vi "Create GB by Co-incident O-lattice.vi"(5 "Skip cleanup?":bool, 6 "Max # of atoms":i32=9999999, 7 "Collision Removal":T1={"Min Seperation Distance (A)"=2.0, "Edge Duplication Range (A)"=3.0}, 8 "Co-incident Tolerance":dbl=0.01, 9 "Number of integers to search":i32=50, 10 "Grain Growth and Geometry":T5={"Min Grain Length (A)"=5.0, "Min Angle from GB plane"=0.0, "GB Overlap Length (A)"=0.0}, 11 "Grain Boundary Definition":T6={"Grain 1 Orientation"=[1.0, 0.6019417241891012, 0.029651947654046266], "Grain 2 Orientation"=[1.0, 0.730727623275494, 0.2205637301176], "Twist Angle (Deg)"=0.0, "Translation Vector"=[0.0, 0.0, 0.0]}) -> (1 "Creation Time":T4={"Time to create primitives"=0, "Time to Grow to Box"=4152, "Time to find subset"=1109, "Time to Cleanup"=1}, 2 "GB Data":string[][](array[string])=[["Grain 1, h", "Grain 1, k", "Grain 1, L", "Grain 2, h", "Grain 2, k", "Grain 2, L", "Twist Angle (Deg)", "Translation Tx", "Translation Ty", "Translation Tz", "Tilt Angle (Deg)", "Viewing Angle, h", "Viewing Angle, k", "Viewing Angle, L", "Grain 1 Length (factor)", "Grain 2 Length (factor", "Max Grain Height (A)", "Max Grain Width (A)", "Grain 1 Start", "Overlap Region (A)", "Reduction Slab X", "Reduction Slab Y", "Reduction Tolerance (A)", "Min Atomic Separation Distance", "Edge Duplication Range", "# Atoms"], ["1.000000", "0.601942", "0.029652", "1.000000", "0.730728", "0.220564", "0.000000", "0.000000", "0.000000", "0.000000", "10.024930", "1.000000", "-1.661290", "0.000000", "1.000000", "1.000000", "90.000000", "90.000000", "-0.001000", "0.001000", "4.600000", "4.000000", "0.500000", "2.000000", "3.000000", "12135.000000"]], 3 "Grain Boundary":T2={"Structure Name"="(0.00) twist [1.000,0.602,0.030] [1.000,0.731,0.221] (0.00,0.00,0.00)T GB", "Lattice vector a"=[270.03, 0.0, 0.0], "Lattice vector b"=[0.0, 270.03, 0.0], "Lattice vector c"=[0.0, 0.0, 6.006], "Atoms Array"=[{"Atom Name"="Cd", "Positions (Direct)"=array6055x3[18165 elements], "Positions (Cartesian)"=array6055x3[18165 elements]}, {"Atom Name"="Te", "Positions (Direct)"=array6080x3[18240 elements], "Positions (Cartesian)"=array6080x3[18240 elements]}], "# of atoms"=12135} {"Atoms Array"."Positions (Cartesian)" format="%#_4f"; "Atoms Array"."Positions (Direct)" format="%#_4f"})   [LabVIEW 2010]
uses:
  <vilib>/Analysis/baseanly.llb/Real A x B.vi
  <vilib>/Analysis/NI_AALPro.lvlib
  <vilib>/Analysis/NI_AALBase.lvlib
panel:
  in  "GB Plane 1, Lattice a":dbl[](array[numeric])
  in  "GB Plane 2, Lattice b":dbl[](array[numeric])
  in  "Perpendicular to GB Plane, Lattice c":dbl[](array[numeric])
  in  "Conventional Unit Cell":T2={"Structure Name"="CdTe", "Lattice vector a"=[6.615785553057252, 0.0, 0.0], "Lattice vector b"=[0.0, 6.615785553057252, 0.0], "Lattice vector c"=[0.0, 0.0, 6.615785553057252], "Atoms Array"=[{"Atom Name"="Cd", "Positions (Direct)"=[[0.0, 0.0, 0.0], [0.0, 0.5, 0.5], [0.5, 0.0, 0.5], [0.5, 0.5, 0.0]], "Positions (Cartesian)"=[[0.0, 0.0, 0.0], [0.0, 3.307892776528626, 3.307892776528626], [3.307892776528626, 0.0, 3.307892776528626], [3.307892776528626, 3.307892776528626, 0.0]]}, {"Atom Name"="Te", "Positions (Direct)"=[[0.25, 0.25, 0.25], [0.75, 0.75, 0.25], [0.75, 0.25, 0.75], [0.25, 0.75, 0.75]], "Positions (Cartesian)"=[[1.653946388264313, 1.653946388264313, 1.653946388264313], [4.96183916479294, 4.96183916479294, 1.653946388264313], [4.96183916479294, 1.653946388264313, 4.96183916479294], [1.653946388264313, 4.96183916479294, 4.96183916479294]]}], "# of atoms"=8}
  in  "GB Geometry":T3(radio)=enum."Best Triclinic"
  out "error out":errorcluster
  out "Expected # of Atoms":i32=166
  in  "Headers":string[](array[string])=["Grain 1, h", "Grain 1, k", "Grain 1, L", "Grain 2, h", "Grain 2, k", "Grain 2, L", "Twist Angle (Deg)", "Translation Tx", "Translation Ty", "Translation Tz", "Tilt Angle (Deg)", "Viewing Angle, h", "Viewing Angle, k", "Viewing Angle, L", "Grain 1 Length (factor)", "Grain 2 Length (factor", "Max Grain Height (A)", "Max Grain Width (A)", "Grain 1 Start", "Overlap Region (A)", "Reduction Slab X", "Reduction Slab Y", "Reduction Tolerance (A)", "Min Atomic Separation Distance", "Edge Duplication Range", "# Atoms"]
  out "Time to Cleanup":u32=1
  out "Time to find subset":u32=1109
  out "Time to Grow to Box":u32=4152
  out "Time to create primitives":u32
  out "Tilt Angle":dbl=10.024929742348679
  out "# of Atoms Removed":i32=28
  out "Mutual Viewing Angle":dbl[](array[numeric])=[1.0, -1.6612903871170226, 0.0]
  in  "Primitive Unit Cell":T2={"Structure Name"="CdTe", "Lattice vector a"=[6.615785553057252, 0.0, 0.0], "Lattice vector b"=[0.0, 6.615785553057252, 0.0], "Lattice vector c"=[0.0, 0.0, 6.615785553057252], "Atoms Array"=[{"Atom Name"="Cd", "Positions (Direct)"=[[0.0, 0.0, 0.0], [0.0, 0.5, 0.5], [0.5, 0.0, 0.5], [0.5, 0.5, 0.0]], "Positions (Cartesian)"=[[0.0, 0.0, 0.0], [0.0, 3.307892776528626, 3.307892776528626], [3.307892776528626, 0.0, 3.307892776528626], [3.307892776528626, 3.307892776528626, 0.0]]}, {"Atom Name"="Te", "Positions (Direct)"=[[0.25, 0.25, 0.25], [0.75, 0.75, 0.25], [0.75, 0.25, 0.75], [0.25, 0.75, 0.75]], "Positions (Cartesian)"=[[1.653946388264313, 1.653946388264313, 1.653946388264313], [4.96183916479294, 4.96183916479294, 1.653946388264313], [4.96183916479294, 1.653946388264313, 4.96183916479294], [1.653946388264313, 4.96183916479294, 4.96183916479294]]}], "# of atoms"=8}
  # "Remove Collisions"
  # "Primitives"
  # "Grain Growth"
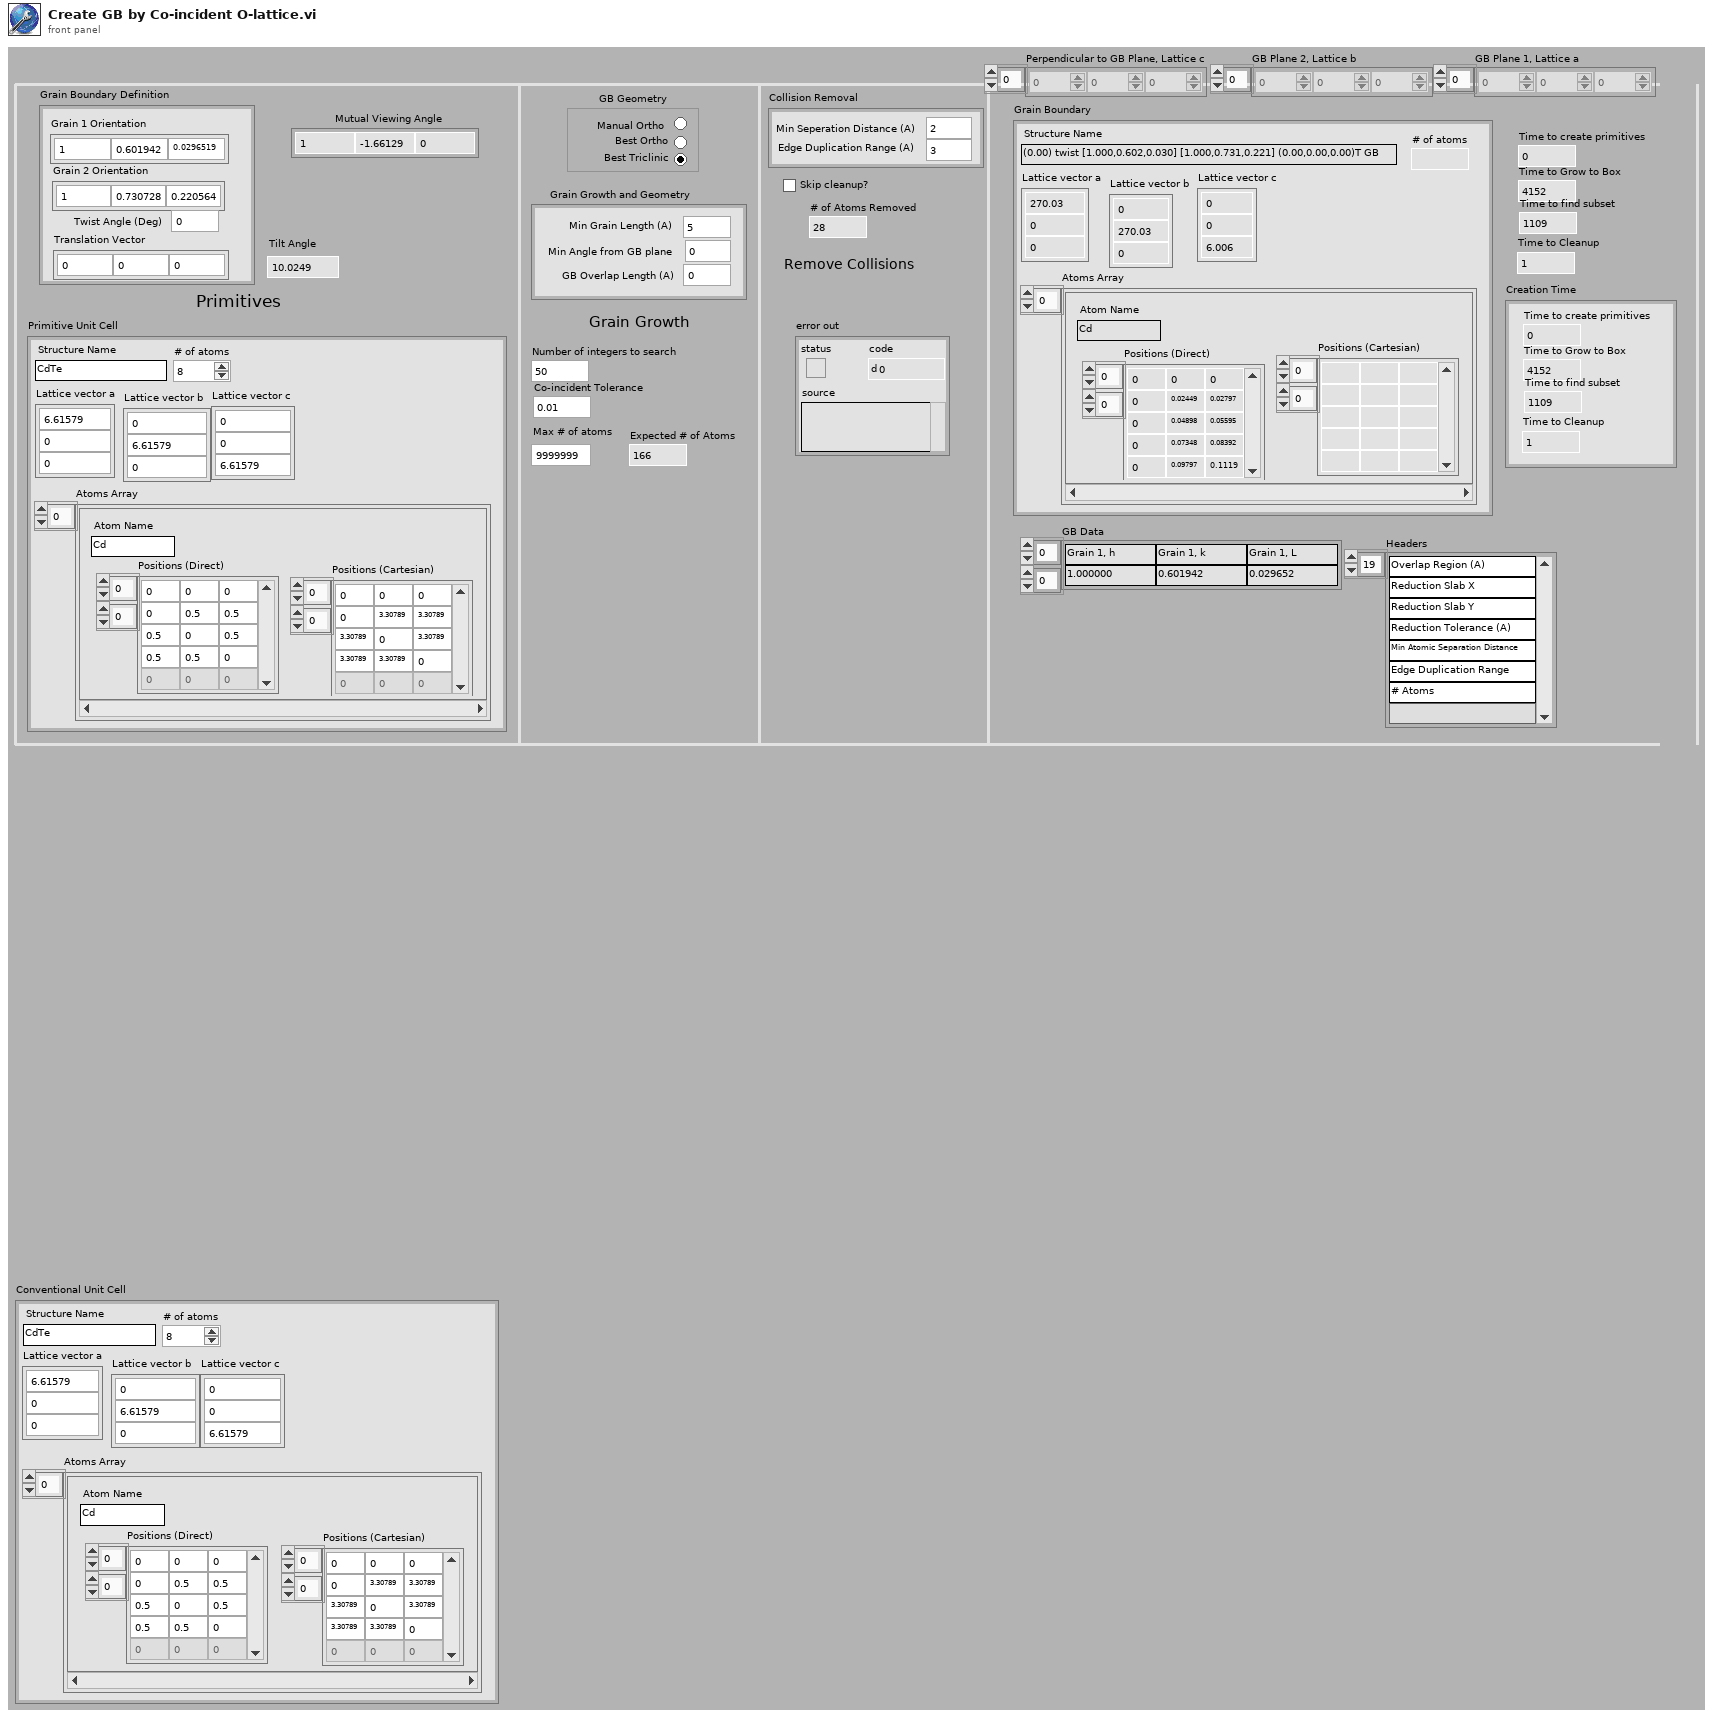
[diagram p1: front panel]
types:
  T1 = cluster{"Min Seperation Distance (A)":dbl, "Edge Duplication Range (A)":dbl}
  T2 = cluster{"Structure Name":string, "Lattice vector a":dbl[], "Lattice vector b":dbl[], "Lattice vector c":dbl[], "Atoms Array":cluster{"Atom Name":string, "Positions (Direct)":dbl[][], "Positions (Cartesian)":dbl[][]}[], "# of atoms":i32}
  T3 = enum32{"Manual Ortho", "Best Ortho", "Best Triclinic"}
  T4 = cluster{"Time to create primitives":u32, "Time to Grow to Box":u32, "Time to find subset":u32, "Time to Cleanup":u32}
  T5 = cluster{"Min Grain Length (A)":dbl, "Min Angle from GB plane":dbl, "GB Overlap Length (A)":dbl}
  T6 = cluster{"Grain 1 Orientation":dbl[], "Grain 2 Orientation":dbl[], "Twist Angle (Deg)":dbl, "Translation Vector":dbl[]}
  T7 = cluster{"Grain 1 Orientation":dbl[], "Grain 2 Orientation":dbl[], "Twist Angle (Deg)":dbl}
  T8 = typedef "NI_Matrix.lvlib/RealMatrix.ctl" = dbl[][]
  T9 = cluster{"Atom Name":string, "Positions (Direct)":dbl[][], "Positions (Cartesian)":dbl[][]}[]
  T10 = cluster{"Atom Name":string, "Positions (Direct)":dbl[][], "Positions (Cartesian)":dbl[][]}
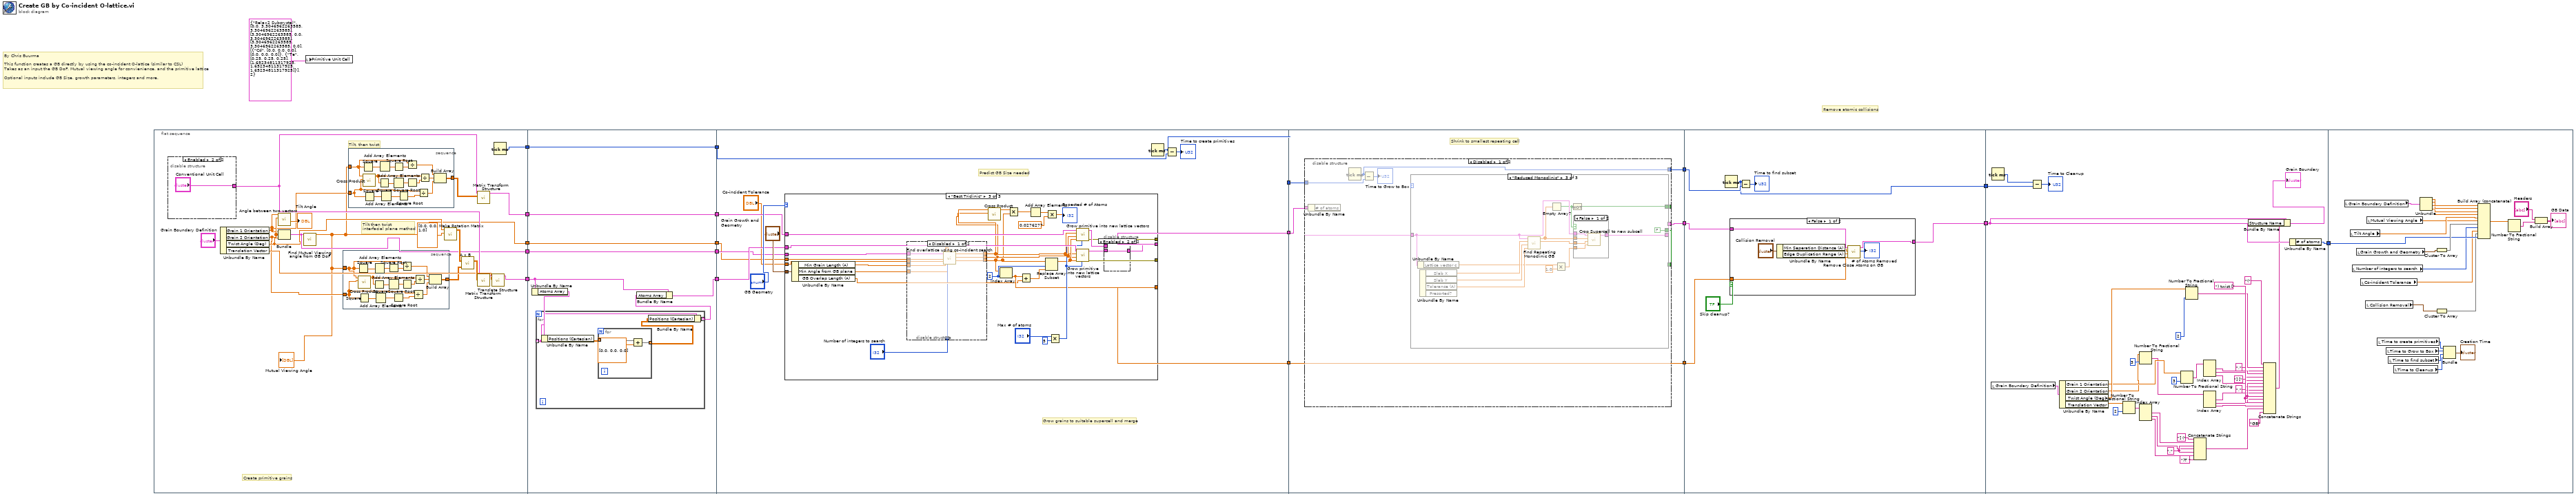
[diagram p0: block diagram]
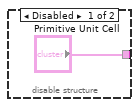
[diagram p2: hidden frame]
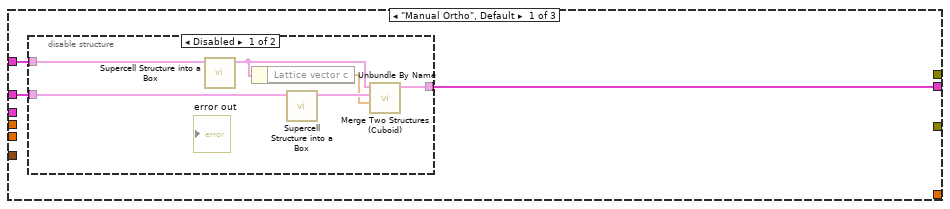
[diagram p3: hidden frame]
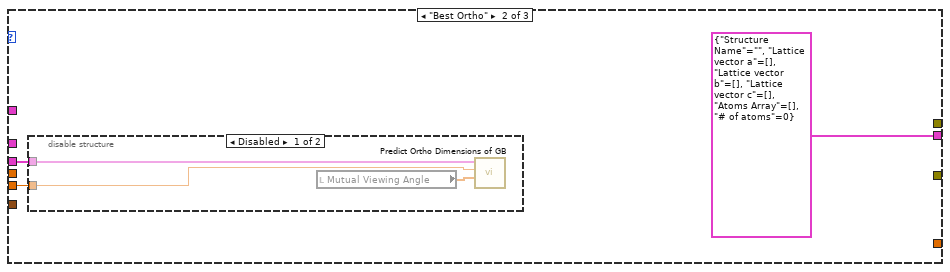
[diagram p5: hidden frame]
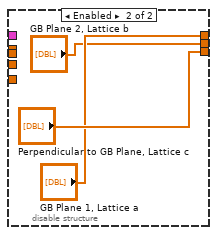
[diagram p7: hidden frame]
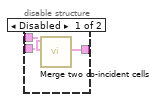
[diagram p8: hidden frame]
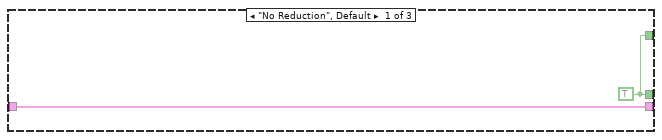
[diagram p9: hidden frame]
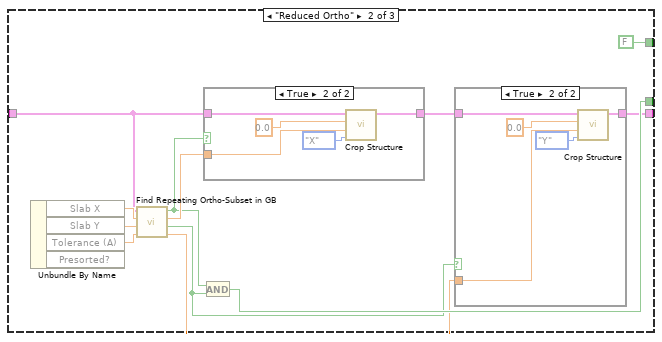
[diagram p10: hidden frame]
diagram:
  # "By Chris Buurma\n\nThis function creates a GB directly by using the co-incident O-lattice (similar to CSL)\nTakes as an input the GB DoF, Mutual viewing angle for convienience, and the primitive lattice\n\nOptional inputs include GB Size, growth parameters, integers and more."
  # "Remove atomic collisions"
  n1 = flat-sequence {
    tunnel: [w34] -> w10
    tunnel: [w38] -> w8
    tunnel: [w31] -> w6
    tunnel: [w22] -> w4
    tunnel: [w27] -> w2
    tunnel: w10 -> [w75]
    tunnel: [w73] -> w9
    tunnel: w8 -> [w80]
    tunnel: [w80] -> w7
    tunnel: w6 -> [w79]
    tunnel: [w79] -> w5
    tunnel: w4 -> [w78]
    tunnel: [w78] -> w3
    tunnel: w2 -> [w77]
    tunnel: [w77] -> w1
    tunnel: w9 -> [w92]
    tunnel: w7 -> [w93]
    tunnel: w5 -> [w97]
    tunnel: w3 -> [w89]
    tunnel: [w98] -> w15
    tunnel: [w96] -> w14
    tunnel: w1 -> [w90]
    tunnel: [w88] -> w11
    tunnel: [w164] -> w18
    tunnel: [w165] -> w17
    tunnel: w14 -> [w162]
    tunnel: w15 -> [w163]
    tunnel: [w161] -> w12
    tunnel: w11 -> [w161]
    tunnel: w18 -> [w226]
    tunnel: [w225] -> w20
    tunnel: w17 -> [w223]
    tunnel: [w222] -> w19
    tunnel: w12 -> [w221]
    tunnel: w20 -> [w246]
    tunnel: w19 -> [w247]
    tunnel: [w245] -> w16
    tunnel: w16 -> [w289]
    frame #0 {
      # "Tilt then twist\ninterfacial plane method"
      # "Tilt, then twist"
      # "Create primitive grains"
      n2 = disable-structure shown="Enabled" {
        disable-tunnel: ["Primitive Unit Cell" "Conventional Unit Cell"] -> w30
        frame Disabled {
        }
        frame Enabled {
        }
      }
      n3 = Unbundle By Name("Grain Boundary Definition") -> ("Grain 1 Orientation"=w23:dbl[], "Grain 2 Orientation"=w25:dbl[], "Twist Angle (Deg)"=w28:dbl, "Translation Vector"=w32:dbl[])
      n4 = call "Angle between two vectors.vi"("Vector 2"=w25, "Vector 1"=w23) -> ("Angle (Degrees)"=→"Tilt Angle":dbl)  [unwired: 7 in, 2 out]
      n5 = Bundle("Grain 1 Orientation"=w23, "Grain 2 Orientation"=w25, "Twist Angle (Deg)"=w28) -> (w27:T7)  [unwired: 1 in]
      n6 = call "Find Mutual Viewing angle from GB DoF.vi"("Grain Boundary Macro DoF"=w27) -> ("Mutual Viewing Angle"=w22:dbl[])  [unwired: 8 in, 2 out]
      "Mutual Viewing Angle" <- w22
      n7 = stacked-sequence {
        tunnel: [w59] -> w24
        tunnel: w25 -> [w58]
        tunnel: w22 -> [w57]
        frame #0 {
          n8 = Square(x=w57) -> (x^2=w66:dbl[])
          n9 = call <vilib>:"Cross Product.vi"("B Vector"=w58, "A Vector"=w57) -> ("Cross Product"=w61:dbl[])  [unwired: 8 in, 1 out]
          n10 = Square(x=w58) -> (x^2=w70:dbl[])
          n11 = Square(x=w61) -> (x^2=w63:dbl[])
          n12 = Add Array Elements(numeric array=w66) -> (sum=w67:dbl)
          n13 = Add Array Elements(numeric array=w70) -> (sum=w69:dbl)
          n14 = Square Root(x=w67) -> (sqrt(x)=w64:dbl)
          n15 = Add Array Elements(numeric array=w63) -> (sum=w62:dbl)
          n16 = Square Root(x=w69) -> (sqrt(x)=w68:dbl)
          n17 = Divide(x=w57, y=w64) -> (x/y=w65:dbl[])
          n18 = Square Root(x=w62) -> (sqrt(x)=w60:dbl)
          n19 = Divide(x=w58, y=w68) -> (x/y=w72:dbl[])
          n20 = Divide(x=w61, y=w60) -> (x/y=w71:dbl[])
          n21 = Build Array(w65, w71, w72) -> (w59:T8)
        }
      }
      n22 = stacked-sequence {
        tunnel: [w43] -> w21
        tunnel: w23 -> [w42]
        tunnel: w22 -> [w41]
        frame #0 {
          n23 = Square(x=w41) -> (x^2=w50:dbl[])
          n24 = call <vilib>:"Cross Product.vi"("B Vector"=w42, "A Vector"=w41) -> ("Cross Product"=w45:dbl[])  [unwired: 8 in, 1 out]
          n25 = Square(x=w42) -> (x^2=w54:dbl[])
          n26 = Square(x=w45) -> (x^2=w47:dbl[])
          n27 = Add Array Elements(numeric array=w50) -> (sum=w51:dbl)
          n28 = Add Array Elements(numeric array=w54) -> (sum=w53:dbl)
          n29 = Square Root(x=w51) -> (sqrt(x)=w48:dbl)
          n30 = Add Array Elements(numeric array=w47) -> (sum=w46:dbl)
          n31 = Square Root(x=w53) -> (sqrt(x)=w52:dbl)
          n32 = Divide(x=w41, y=w48) -> (x/y=w49:dbl[])
          n33 = Square Root(x=w46) -> (sqrt(x)=w44:dbl)
          n34 = Divide(x=w42, y=w52) -> (x/y=w56:dbl[])
          n35 = Divide(x=w45, y=w44) -> (x/y=w55:dbl[])
          n36 = Build Array(w49, w55, w56) -> (w43:T8)
        }
      }
      n37 = call "Make Rotation Matrix.vi"("Rotation Axis"=dbl[] [0.0, 0.0, 1.0], "Rotation Angle (Degree)"=w28) -> ("Rotation Matrix"=w36:T8)  [unwired: 9 in]
      n38 = call-poly <vilib>:"A x B.vi"("B"=w24, "A"=w36) -> ("A x B"=w35:T8)  [unwired: 1 out]
      n39 = call "Matrix Transform Structure.vi"("Matrix Transform"=w21, "Original Structure"=w30) -> ("After Transform"=w38:T2)  [unwired: 9 in]
      n40 = call "Matrix Transform Structure.vi"("Matrix Transform"=w35, "Original Structure"=w30) -> ("After Transform"=w37:T2)  [unwired: 9 in]
      n41 = call "Translate Structure.vi"("Translation Vector (Cartesian)"=w32, "Atomic Structure"=w37) -> ("Shifted Structure"=w34:T2)  [unwired: 9 in]
      n42 = Tick Count (ms)() -> (millisecond timer value=w31:u32)
    }
    frame #1 {
      n43 = Unbundle By Name(w75) -> ("Atoms Array"=w76:T9)
      n44 = for {
        tunnel: w76 -> [w83] mode=indexing
        tunnel: [w81] -> w74 mode=indexing
        n45 = Unbundle By Name(w83) -> ("Positions (Cartesian)"=w84:dbl[][])
        n46 = for {
          tunnel: w84 -> [w87] mode=indexing
          tunnel: [w85] -> w82 mode=indexing
          n47 = Add(x=w87, y=dbl[] [0.0, 0.0, 0.0]) -> (x+y=w85:dbl[])
        }
        n48 = Bundle By Name(cluster=w83, "Positions (Cartesian)"=w82) -> (w81:T10)
      }
      n49 = Bundle By Name(cluster=w75, "Atoms Array"=w74) -> (w73:T2)
    }
    frame #2 {
      # "Grow grains to suitable supercell and merge"
      # "Predict GB Size needed"
      n50 = case shown="\"Best Triclinic\"" "GB Geometry" {
        tunnel: [w102 T2 {"Structure Name"="", "Lattice vector a"=[], "Lattice vector b"=[], "Lattice vector c"=[], "Atoms Array"=[], "# of atoms"=0} ("Atomic Structure of 1 + 2 by T") w138] -> w98
        tunnel: "Grain Growth and Geometry" -> [_ _ w129]
        tunnel: w93 -> [w101 _ w137]
        tunnel: w92 -> [w100 _ w136]
        tunnel: "Co-incident Tolerance" -> [_ w110 w141]
        tunnel: w90 -> [_ w111 w144]
        tunnel: w89 -> [_ _ w143]
        tunnel: [_ _ w130] -> w88
        tunnel: [_ _ w125] -> _
        tunnel: [_ _ w124] -> _
        frame "Manual Ortho", Default {
          n51 = disable-structure shown="Disabled" {
            disable-tunnel: [w105 _] -> w102
            disable-tunnel: w101 -> [w104 _]
            disable-tunnel: w100 -> [w103 _]
            frame Disabled {
              n52 = call "Supercell Structure into a Box.vi"("Subcrystal"=w104) -> ("Expanded cubic Structure"=w108:T2)  [unwired: 8 in, 2 out]
              n53 = Unbundle By Name(w108) -> ("Lattice vector c"=w106:dbl[])
              n54 = call "Supercell Structure into a Box.vi"("Subcrystal"=w103) -> ("Expanded cubic Structure"=w107:T2)  [unwired: 8 in, 2 out]
              n55 = call "Merge Two Structures (Cuboid).vi"("Translation Vector (1 to 2)"=w106, "Atomic Structure 2"=w107, "Atomic Structure 1"=w108) -> ("Atomic Structure of 1 + 2 by T"=w105:T2)  [unwired: 8 in]
            }
            frame Enabled {
            }
          }
        }
        frame "Best Ortho" {
          n56 = disable-structure shown="Disabled" {
            disable-tunnel: w111 -> [w114 _]
            disable-tunnel: w110 -> [w113 _]
            frame Disabled {
              n57 = local read "Mutual Viewing Angle"() -> (w112:dbl[])
              n58 = call "Predict Ortho Dimensions of GB.vi"("Mutual Viewing Angle"=w112, "Tolerance"=w113, "Grain Boundary Macro Definition"=w114) -> ()  [unwired: 6 in, 3 out]
            }
            frame Enabled {
            }
          }
        }
        frame "Best Triclinic" {
          w132 = 2 ("index")
          n59 = Unbundle By Name(w129) -> ("Min Grain Length (A)"=w127:dbl, "Min Angle from GB plane"=w128:dbl, "GB Overlap Length (A)"=w126:dbl)
          n60 = disable-structure shown="Disabled" {
            disable-tunnel: w144 -> [w153 _]
            disable-tunnel: w143 -> [w152 _]
            disable-tunnel: "Number of integers to search" -> [w151 _]
            disable-tunnel: w141 -> [w150 _]
            disable-tunnel: w128 -> [w149 _]
            disable-tunnel: w127 -> [w148 _]
            disable-tunnel: [w147 "GB Plane 1, Lattice a"] -> w123
            disable-tunnel: [w146 "GB Plane 2, Lattice b"] -> w122
            disable-tunnel: [w145 "Perpendicular to GB Plane, Lattice c"] -> w121
            frame Disabled {
              n61 = call "Find overlattice using co-incident search.vi"("Minimal Angle from GB plane"=w149, "Minimal thickness of the grain (A)"=w148, "Co-incidence Tolerance"=w150, "Number of integers to search"=w151, "Mutual Viewing Angle"=w152, "Grain Boundary Macro Definition"=w153) -> ("Perpendicular to GB Plane, Lattice c"=w145:dbl[], "GB Plane 2, Lattice b"=w146:dbl[], "GB Plane 1, Lattice a"=w147:dbl[])  [unwired: 3 in]
            }
            frame Enabled {
            }
          }
          n62 = call <vilib>:"Cross Product.vi"("B Vector"=w122, "A Vector"=w123) -> ("Cross Product"=w120:dbl[])  [unwired: 8 in, 1 out]
          n63 = Index Array(array=w121, index=w132) -> (element=w130:dbl)
          n64 = Multiply(x=w120, y=w121) -> (x*y=w119:dbl[])
          n65 = Add(x=w130, y=w126) -> (x+y=w115:dbl)
          n66 = Add Array Elements(numeric array=w119) -> (sum=w118:dbl)
          n67 = Replace Array Subset(array=w121, new element=w115, index=w132) -> (w131:dbl[])
          n68 = Multiply(x=w118, y=0.0276277) -> (x*y=→"Expected # of Atoms":dbl)
          n69 = Multiply(x="Max # of atoms", y=5) -> (x*y=w135:i32)
          n70 = call "Grow primitive into new lattice vectors.vi"("Max # of atoms"=w135, "New Lattice Vector c"=w131, "New Lattice Vector b"=w122, "New Lattice Vector a"=w123, "Primitive"=w137) -> ("error out"=w124:errorcluster, "Expanded to new Vectors"=w133:T2)  [unwired: 4 in, 1 out]
          n71 = call "Grow primitive into new lattice vectors.vi"("Max # of atoms"=w135, "New Lattice Vector c"=w131, "New Lattice Vector b"=w122, "New Lattice Vector a"=w123, "Primitive"=w136) -> ("error out"=w125:errorcluster, "Expanded to new Vectors"=w134:T2)  [unwired: 4 in, 1 out]
          n72 = disable-structure shown="Enabled" {
            disable-tunnel: [w159 w160] -> w138
            disable-tunnel: w134 -> [w158 w160]
            disable-tunnel: w133 -> [w157 _]
            frame Disabled {
              n73 = call "Merge two co-incident cells.vi"("Grain 2"=w158, "Grain 1"=w157) -> ("Joined GB"=w159:T2)  [unwired: 9 in]
            }
            frame Enabled {
            }
          }
        }
      }
      n74 = Tick Count (ms)() -> (millisecond timer value=w96:u32)
      n75 = Subtract(x=w96, y=w97) -> (x-y=→"Time to create primitives":u32)
    }
    frame #3 {
      # "Shrink to smallest repeating cell"
      n76 = disable-structure shown="Disabled" {
        disable-tunnel: [w173 _] -> w165
        disable-tunnel: [w172 w219] -> w164
        disable-tunnel: [w171 _] -> _
        disable-tunnel: [w170 _] -> _
        disable-tunnel: w163 -> [w167 w219]
        disable-tunnel: w162 -> [w166 _]
        frame Disabled {
          n77 = Unbundle By Name(w167) -> ("# of atoms"=w168:i32)
          n78 = Tick Count (ms)() -> (millisecond timer value=w173:u32)
          n79 = Subtract(x=w173, y=w166) -> (x-y=→"Time to Grow to Box":u32)
          n80 = case shown="\"Reduced Monoclinic\"" {
            selector: _ -> [_ _ _]
            tunnel: [w175 w177 w202] -> w172
            tunnel: [w174 FALSE w201] -> w171
            tunnel: [w174 w187 FALSE] -> w170
            tunnel: w167 -> [w175 w183 w209]
            frame "No Reduction", Default {
              w174 = TRUE
            }
            frame "Reduced Ortho" {
              n81 = Unbundle By Name() -> ("Slab X"=w186:dbl, "Slab Y"=w185:dbl, "Tolerance (A)"=w184:dbl)  [unwired: 1 in, 1 out]
              n82 = call "Find Repeating Ortho-Subset in GB.vi"("Tolerance (A)"=w184, "Slab Y"=w185, "Slab X"=w186, "Grain Boundary"=w183) -> ("Repeating Y Length Scale"=w180:dbl, "Subset Y found?!"=w178:bool, "Repeating X Length Scale"=w181:dbl, "Subset X found?!"=w179:bool)  [unwired: 4 in]
              n83 = And(x=w179, y=w178) -> (x .and. y?=w187:bool)
              n84 = case shown="True" w179 {
                tunnel: w183 -> [w194 w199]
                tunnel: [w194 w196] -> w182
                tunnel: w181 -> [_ w195]
                frame False {
                }
                frame True {
                  n85 = call "Crop Structure.vi"("Cropping Index"=enum16{"X", "Y", "Z"}."X", "Upper Bound Z"=w195, "Lower bound Z"=0.0, "Input Structure"=w199) -> ("Cropped Structure"=w196:T2)  [unwired: 7 in]
                }
              }
              n86 = case shown="True" w178 {
                tunnel: w182 -> [w188 w193]
                tunnel: w180 -> [_ w191]
                tunnel: [w188 w189] -> w177
                frame False {
                }
                frame True {
                  n87 = call "Crop Structure.vi"("Cropping Index"=enum16{"X", "Y", "Z"}."Y", "Upper Bound Z"=w191, "Lower bound Z"=0.0, "Input Structure"=w193) -> ("Cropped Structure"=w189:T2)  [unwired: 7 in]
                }
              }
            }
            frame "Reduced Monoclinic" {
              n88 = Unbundle By Name(w209) -> ("Lattice vector c"=w206:dbl[])
              n89 = Unbundle By Name() -> ("Slab X"=w212:dbl, "Slab Y"=w211:dbl, "Tolerance (A)"=w210:dbl)  [unwired: 1 in, 1 out]
              n90 = call "Find Repeating Monoclinic GB.vi"("Tolerance (A)"=w210, "Slab Y"=w211, "Slab X"=w212, "Supercell Structure"=w209) -> ("New Lattice Vector b"=w208:dbl[], "New Lattice Vector a"=w204:dbl[])  [unwired: 5 in, 1 out]
              n91 = Empty Array?(array=w204) -> (empty?=w203:bool)
              n92 = Multiply(x=w206, y=1.0) -> (x*y=w205:dbl[])
              n93 = Not(x=w203) -> (.not. x?=w201:bool)
              n94 = case shown="False" w203 {
                tunnel: w208 -> [w217 _]
                tunnel: w204 -> [w216 _]
                tunnel: w205 -> [w215 _]
                tunnel: w209 -> [w214 w218]
                tunnel: [w213 w218] -> w202
                frame False {
                  n95 = call "Crop Supercell to new subcell.vi"("New Lattice Vector c"=w215, "New Lattice Vector b"=w217, "New Lattice Vector a"=w216, "Supercell Structure"=w214) -> ("Reduced Structure"=w213:T2)  [unwired: 7 in]
                }
                frame True {
                }
              }
            }
          }
        }
        frame Enabled {
        }
      }
    }
    frame #4 {
      n96 = Tick Count (ms)() -> (millisecond timer value=w222:u32)
      n97 = case shown="False" "Skip cleanup?" {
        tunnel: w226 -> [w231 w234]
        tunnel: [w232 w234] -> w225
        tunnel: w221 -> [w227 _]
        frame False {
          n98 = Unbundle By Name("Collision Removal") -> ("Min Seperation Distance (A)"=w229:dbl, "Edge Duplication Range (A)"=w228:dbl)
          n99 = call "Remove Close Atoms on GB.vi"("Grain Boundary Location (A)"=w227, "Edge Duplication Range"=w228, "Minimally Allowable Distance (A)"=w229, "Structure"=w231) -> ("# of Atoms Removed"=→"# of Atoms Removed":i32, "Structure with atoms removed"=w232:T2)  [unwired: 6 in]
        }
        frame True {
        }
      }
      n100 = Subtract(x=w222, y=w223) -> (x-y=→"Time to find subset":u32)
    }
    frame #5 {
      w268 = "," ("string")
      w261 = "," ("string")
      n101 = local read "Grain Boundary Definition"() -> (w271:T6)
      n102 = Tick Count (ms)() -> (millisecond timer value=w248:u32)
      n103 = Subtract(x=w248, y=w247) -> (x-y=→"Time to Cleanup":u32)
      n104 = Unbundle By Name(w271) -> ("Grain 1 Orientation"=w242:dbl[], "Grain 2 Orientation"=w239:dbl[], "Twist Angle (Deg)"=w272:dbl, "Translation Vector"=w273:dbl[])
      n105 = Number To Fractional String(number=w273, precision (6)=i16 2) -> (F-format string=w264:string[])  [unwired: 2 in]
      n106 = Number To Fractional String(number=w239, precision (6)=i16 3) -> (F-format string=w238:string[])  [unwired: 2 in]
      n107 = Index Array(array=w264) -> (element #1=w265:string, element #2=w267:string, element #3=w269:string)  [unwired: 3 in]
      n108 = Number To Fractional String(number=w242, precision (6)=i16 3) -> (F-format string=w241:string[])  [unwired: 2 in]
      n109 = Number To Fractional String(number=w272, precision (6)=i16 2) -> (F-format string=w252:string)  [unwired: 2 in]
      n110 = Concatenate Strings("] (" ("string"), w265, w268, w267, w268, w269, ")T " ("string")) -> (w237:string)
      n111 = Index Array(array=w241) -> (element #1=w254:string, element #2=w256:string, element #3=w257:string)  [unwired: 3 in]
      n112 = Index Array(array=w238) -> (element #1=w259:string, element #2=w260:string, element #3=w262:string)  [unwired: 3 in]
      n113 = Concatenate Strings("(" ("string"), w252, ") twist [" ("string"), w254, "," ("string"), w256, w261, w257, "] [" ("string"), w259, w261, w260, w261, w262, w237, "GB" ("string")) -> (w235:string)
      n114 = Bundle By Name(cluster=w246, "Structure Name"=w235) -> (→"Grain Boundary":T2)
      n115 = Unbundle By Name(w246) -> ("# of atoms"=w245:i32)
    }
    frame #6 {
      n116 = local read "Grain Boundary Definition"() -> (w296:T6)
      n117 = local read "Tilt Angle"() -> (w285:dbl)
      n118 = local read "Number of integers to search"() -> (w277:i32)
      n119 = local read "Grain Growth and Geometry"() -> (w291:T5)
      n120 = local read "Co-incident Tolerance"() -> (w276:dbl)
      n121 = local read "Collision Removal"() -> (w275:T1)
      n122 = local read "Mutual Viewing Angle"() -> (w284:dbl[])
      n123 = local read "Time to create primitives"() -> (w281:u32)
      n124 = local read "Time to Grow to Box"() -> (w280:u32)
      n125 = local read "Time to find subset"() -> (w279:u32)
      n126 = local read "Time to Cleanup"() -> (w282:u32)
      n127 = Unbundle(w296) -> ("Grain 1 Orientation"=w295:dbl[], "Grain 2 Orientation"=w294:dbl[], "Twist Angle (Deg)"=w293:dbl, "Translation Vector"=w292:dbl[])
      n128 = Cluster To Array(cluster=w291) -> (array=w290:dbl[])
      n129 = Cluster To Array(cluster=w275) -> (array=w274:dbl[])
      n130 = Bundle("Time to create primitives"=w281, "Time to Grow to Box"=w280, "Time to find subset"=w279, "Time to Cleanup"=w282) -> (→"Creation Time":T4)  [unwired: 1 in]
      n131 = Build Array (concatenate)(w295, w294, w293, w292, w285, w284, w290, w277, w276, w274, w289) -> (w288:dbl[])
      n132 = Number To Fractional String(number=w288) -> (F-format string=w287:string[])  [unwired: 3 in]
      n133 = Build Array("Headers", w287) -> (→"GB Data":string[][])
    }
  }
  n134 = local write "Primitive Unit Cell"(T2 {"Structure Name"="Relax2 Subcrystal", "Lattice vector a"=[0.0, 3.3046962263585, 3.3046962263585], "Lattice vector b"=[3.3046962263585, 0.0, 3.3046962263585], "Lattice vector c"=[3.3046962263585, 3.3046962263585, 0.0], "Atoms Array"=[{"Atom Name"="Cd", "Positions (Direct)"=[[0.0, 0.0, 0.0]], "Positions (Cartesian)"=[[0.0, 0.0, 0.0]]}, {"Atom Name"="Te", "Positions (Direct)"=[[0.25, 0.25, 0.25]], "Positions (Cartesian)"=[[1.65234811317925, 1.65234811317925, 1.65234811317925]]}], "# of atoms"=2} ("Primitive Lattice Vectors")) -> ()
